vi "SCM PS Control Remote2.vi"() -> ()   [LabVIEW 2025]
panel:
  out "x = y?":bool
  in  "Hold":bool
  out "error out 3":errorcluster={"status"=TRUE, "code"=1055, "source"="Close Reference in SCM PS Control Remote2.vi"}
  in  "menu":T1(ring)
  in  "Slew Rate [T/min]":dbl=0.2 format="%#_4g"
  in  "Setpoint [T]":dbl format="%#_4g"
  in  "stop":bool
  in  "port":u16=3375
  in  "error in (no error) 2":errorcluster
  in  "Data mac ip address":string="146.201.200.173"
  out "Field [T]":dbl format="%#_4g"
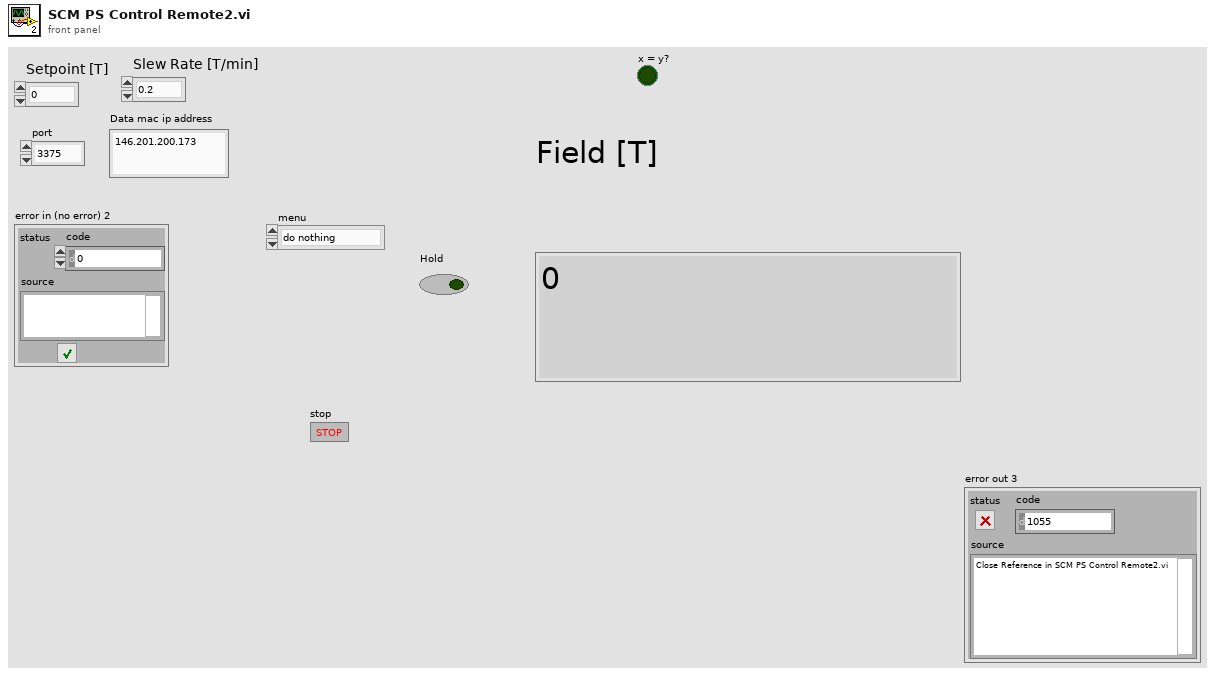
[diagram p1: front panel]
types:
  T1 = enum16{"do nothing", "Ramp To Setpoint", "change set point", "change slew rate"}
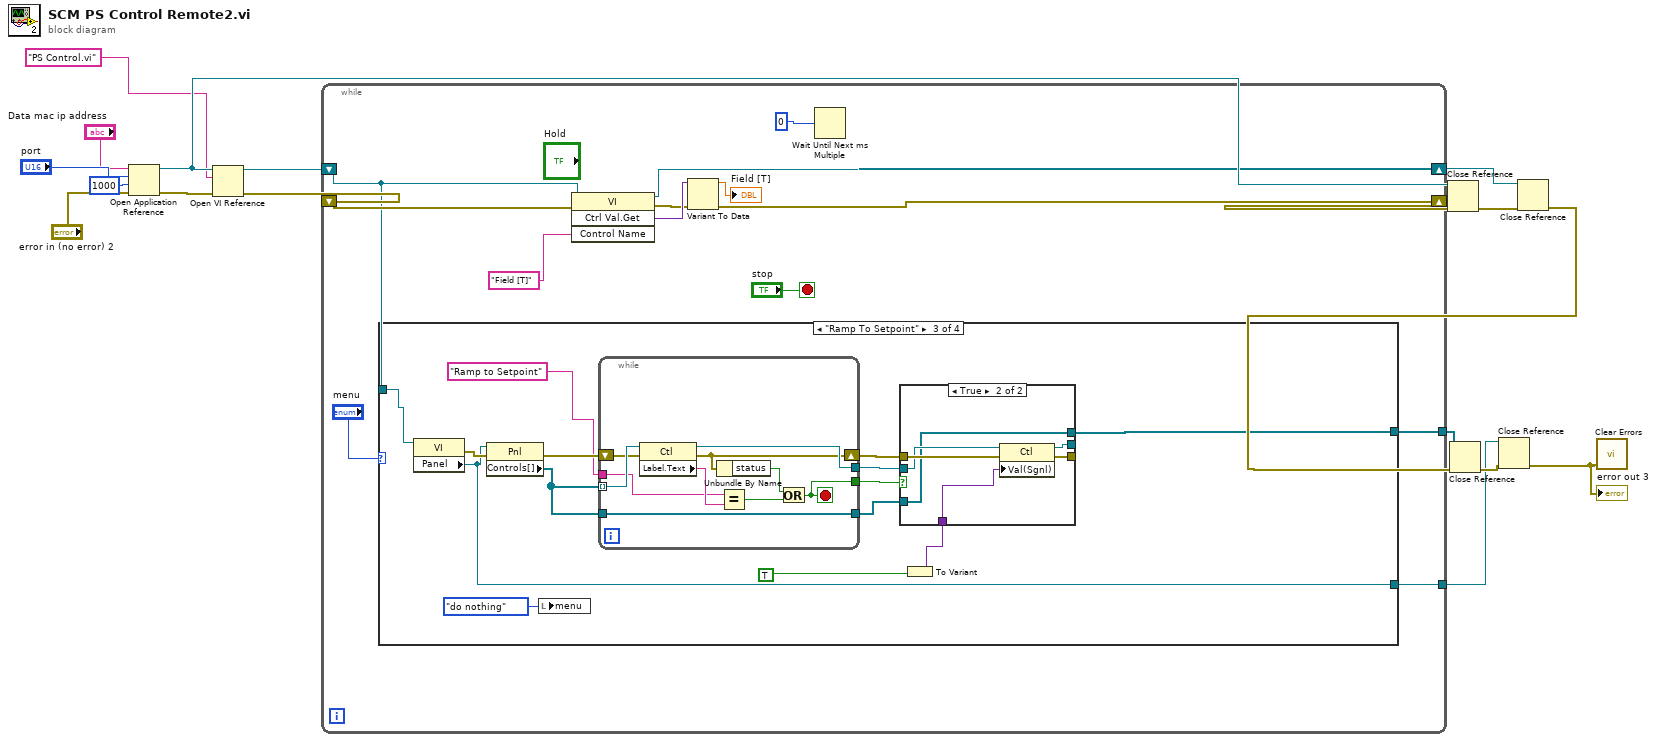
[diagram p0: block diagram]
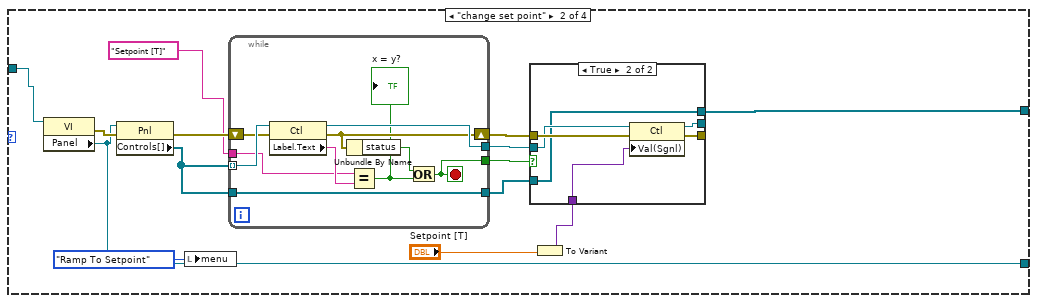
[diagram p3: hidden frame]
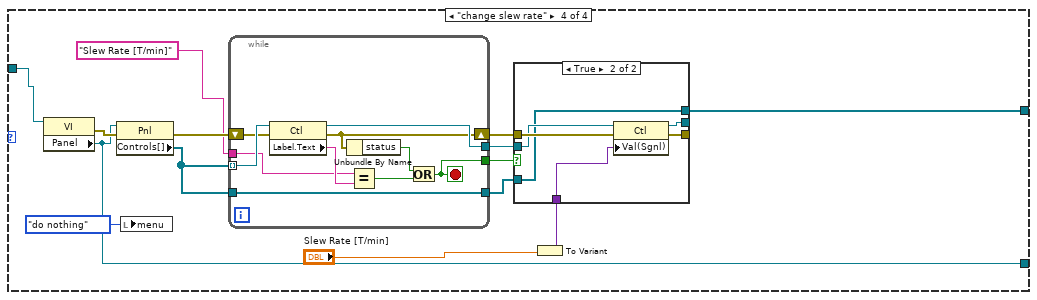
[diagram p6: hidden frame]
diagram:
  n1 = Open Application Reference(8:"error in (no error) 2", 9:1000 ("timeout ms (60000)"), 10:"port", 11:"Data mac ip address") -> (0:w16:errorcluster, 3:w10:refnum<vi>)
  n2 = Open VI Reference(application reference (local)=w10, vi path="PS Control.vi" ("VI name"), error in (no error)=w16) -> (vi reference=w8:refnum<vi>, error out=w13:errorcluster)  [unwired: 3 in]
  n3 = while {
    shift-right: [w28] -> w9
    shift-left: w8 -> [w21]
    shift-right: [w30] -> w12
    shift-left: w13 -> [w24]
    tunnel: [w19] -> w5
    tunnel: [w18] -> w4
    stop <- "stop" stop-if-true
    n4 = case shown="\"Ramp To Setpoint\"" "menu" {
      tunnel: w21 -> [_ w34 w68 w101]
      tunnel: [_ w33 w67 w99] -> w19
      tunnel: [_ w32 w66 w98] -> w18
      frame "do nothing", Default {
      }
      frame "change set point" {
        n5 = property class="VI"(reference=w34) -> (error out=w43:errorcluster, "Panel"=w32:refnum<vi>)  [unwired: 1 in, 1 out]
        n6 = property class="Pnl"(reference=w32, error in=w43) -> (error out=w42:errorcluster, "Controls[]"=w44:refnum<vi>[])  [unwired: 1 out]
        n7 = local write "menu"(T1."Ramp To Setpoint" ("menu")) -> ()
        n8 = while {
          tunnel: w44 -> [w63] mode=indexing
          tunnel: "Setpoint [T]" ("Control Name") -> [w61]
          shift-right: [w58] -> w39
          shift-left: w42 -> [w60]
          tunnel: [w59] -> w41
          tunnel: [w55] -> w40
          tunnel: w44 -> [w54]
          tunnel: [w54] -> w38
          stop <- w55 stop-if-true
          n9 = property class="Ctl"(reference=w63, error in=w60) -> (reference out=w59:refnum<vi>, error out=w58:errorcluster, "Label.Text"=w62:string)
          n10 = Unbundle By Name(w58) -> ("status"=w57:bool)
          n11 = Equal?(x=w61, y=w62) -> (x = y?=w56:bool)
          "x = y?" <- w56
          n12 = Or(x=w57, y=w56) -> (x .or. y?=w55:bool)
        }
        n13 = To Variant(anything="Setpoint [T]") -> (Variant=w36:variant)
        n14 = case shown="True" w40 {
          tunnel: w41 -> [w46 w52]
          tunnel: w39 -> [w47 w53]
          tunnel: [w47 w51] -> _
          tunnel: [w46 w50] -> _
          tunnel: w38 -> [w45 w49]
          tunnel: [w45 w49] -> w33
          tunnel: w36 -> [_ w48]
          frame False {
          }
          frame True {
            n15 = property class="Ctl"(reference=w52, error in=w53, "Val(Sgnl)"=w48) -> (reference out=w50:refnum<vi>, error out=w51:errorcluster)
          }
        }
      }
      frame "Ramp To Setpoint" {
        n16 = property class="VI"(reference=w68) -> (error out=w76:errorcluster, "Panel"=w66:refnum<vi>)  [unwired: 1 in, 1 out]
        n17 = property class="Pnl"(reference=w66, error in=w76) -> (error out=w75:errorcluster, "Controls[]"=w77:refnum<vi>[])  [unwired: 1 out]
        n18 = local write "menu"(T1."do nothing" ("menu")) -> ()
        n19 = while {
          tunnel: w77 -> [w96] mode=indexing
          tunnel: "Ramp to Setpoint" ("Control Name") -> [w94]
          shift-right: [w91] -> w72
          shift-left: w75 -> [w93]
          tunnel: [w92] -> w74
          tunnel: [w88] -> w73
          tunnel: w77 -> [w87]
          tunnel: [w87] -> w71
          stop <- w88 stop-if-true
          n20 = property class="Ctl"(reference=w96, error in=w93) -> (reference out=w92:refnum<vi>, error out=w91:errorcluster, "Label.Text"=w95:string)
          n21 = Unbundle By Name(w91) -> ("status"=w90:bool)
          n22 = Equal?(x=w94, y=w95) -> (x = y?=w89:bool)
          n23 = Or(x=w90, y=w89) -> (x .or. y?=w88:bool)
        }
        n24 = To Variant(anything=TRUE) -> (Variant=w69:variant)
        n25 = case shown="True" w73 {
          tunnel: w74 -> [w79 w85]
          tunnel: w72 -> [w80 w86]
          tunnel: [w80 w84] -> _
          tunnel: [w79 w83] -> _
          tunnel: w71 -> [w78 w82]
          tunnel: [w78 w82] -> w67
          tunnel: w69 -> [_ w81]
          frame False {
          }
          frame True {
            n26 = property class="Ctl"(reference=w85, error in=w86, "Val(Sgnl)"=w81) -> (reference out=w83:refnum<vi>, error out=w84:errorcluster)
          }
        }
      }
      frame "change slew rate" {
        n27 = property class="VI"(reference=w101) -> (error out=w109:errorcluster, "Panel"=w98:refnum<vi>)  [unwired: 1 in, 1 out]
        n28 = property class="Pnl"(reference=w98, error in=w109) -> (error out=w108:errorcluster, "Controls[]"=w110:refnum<vi>[])  [unwired: 1 out]
        n29 = local write "menu"(T1."do nothing" ("menu")) -> ()
        n30 = while {
          tunnel: w110 -> [w129] mode=indexing
          tunnel: "Slew Rate [T/min]" ("Control Name") -> [w127]
          shift-right: [w124] -> w105
          shift-left: w108 -> [w126]
          tunnel: [w125] -> w107
          tunnel: [w121] -> w106
          tunnel: w110 -> [w120]
          tunnel: [w120] -> w104
          stop <- w121 stop-if-true
          n31 = property class="Ctl"(reference=w129, error in=w126) -> (reference out=w125:refnum<vi>, error out=w124:errorcluster, "Label.Text"=w128:string)
          n32 = Unbundle By Name(w124) -> ("status"=w123:bool)
          n33 = Equal?(x=w127, y=w128) -> (x = y?=w122:bool)
          n34 = Or(x=w123, y=w122) -> (x .or. y?=w121:bool)
        }
        n35 = To Variant(anything="Slew Rate [T/min]") -> (Variant=w102:variant)
        n36 = case shown="True" w106 {
          tunnel: w107 -> [w112 w118]
          tunnel: w105 -> [w113 w119]
          tunnel: [w113 w117] -> _
          tunnel: [w112 w116] -> _
          tunnel: w104 -> [w111 w115]
          tunnel: [w111 w115] -> w99
          tunnel: w102 -> [_ w114]
          frame False {
          }
          frame True {
            n37 = property class="Ctl"(reference=w118, error in=w119, "Val(Sgnl)"=w114) -> (reference out=w116:refnum<vi>, error out=w117:errorcluster)
          }
        }
      }
    }
    n38 = invoke class="VI" method="Ctrl Val.Get"(reference=w21, error in=w24, "Control Name"="Field [T]") -> (reference out=w28:refnum<vi>, error out=w26:errorcluster, "Get Control Value Variant"=w27:variant)  [unwired: 1 in, 1 out]
    n39 = Variant To Data(error in=w26, Variant=w27) -> (data=→"Field [T]":dbl, error out=w30:errorcluster)  [unwired: 1 in]
    n40 = Wait Until Next ms Multiple(millisecond multiple=u32 0) -> ()  [unwired: 1 out]
  }
  n41 = Close Reference(reference=w10, error in (no error)=w12) -> (error out=w11:errorcluster)
  n42 = Close Reference(reference=w9, error in (no error)=w11) -> (error out=w2:errorcluster)
  n43 = Close Reference(reference=w5, error in (no error)=w2) -> (error out=w6:errorcluster)
  n44 = Close Reference(reference=w4, error in (no error)=w6) -> (error out=w3:errorcluster)
  "error out 3" <- w3
  n45 = call <vilib>:"Clear Errors.vi"("error in (no error)"=w3) -> ()  [unwired: 5 in, 2 out]
